vi "Image in Header or Footer.vi"(0 "report in":refnum<class "NI_HTML.lvclass">, 5 "select header or footer":u16(ring) items=["Left Header", "Left Footer", "Center Header", "Center Footer", "Right Herader", "Right Footer"], 9 "image path":string, 11 "error in (no error)":errorcluster, 12 "text above image":string) -> (4 "report out":refnum<class "NI_HTML.lvclass">, 15 "error out":errorcluster)   [LabVIEW 2017, in "NI_HTML.lvclass"]
doc: "This VI sets an image for the report header or footer.\n\nRemember, with the HTML report type the left, center, and right header texts are placed on separate lines."
uses:
  <vilib>/Utility/NIReport.llb/HTML/NI_HTML.lvclass
  <vilib>/Utility/NIReport.llb/HTML/NI_HTML.lvclass/NI_HTML.ctl
  <vilib>/Utility/NIReport.llb/NI_ReportGenerationCore.lvlib
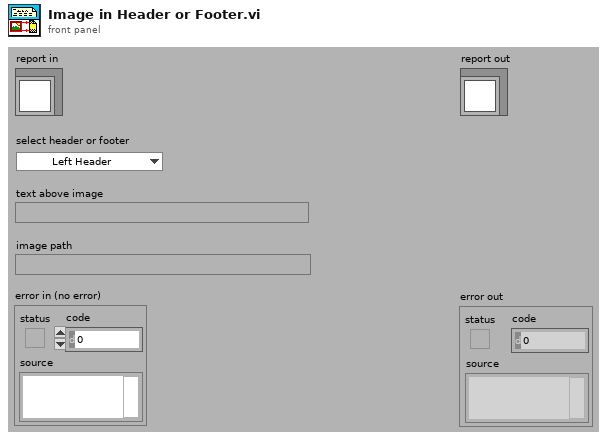
[diagram p1: front panel]
types:
  T1 = typedef "NI_ReportGenerationCore.lvlib/HTML Report Data.ctl" = cluster{"Body Text":string, "Font Tag":string, "Title Text":string, "Header Text":string, "Footer Text":string, "Image List":path[]}
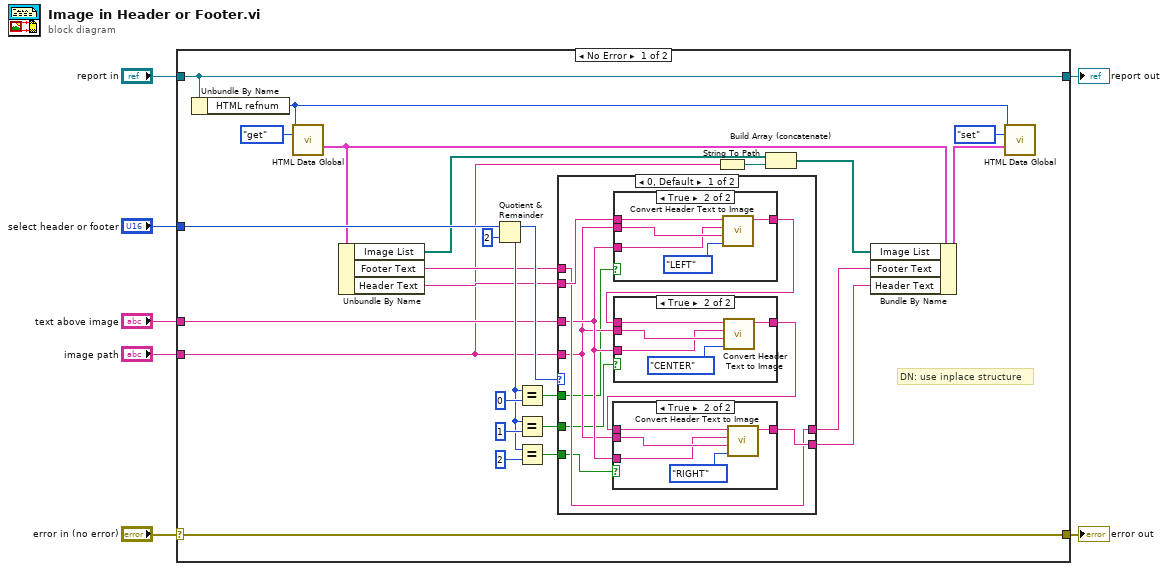
[diagram p0: block diagram]
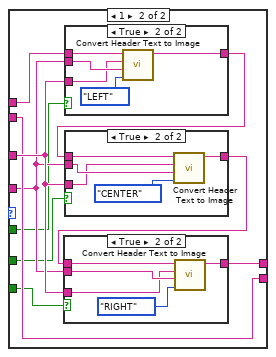
[diagram p5: hidden frame]
diagram:
  n1 = case shown="No Error" "error in (no error)" {
    selector: "error in (no error)" -> [w33 w91]
    tunnel: [w33 w91] -> w6
    tunnel: [w11 w90] -> w4
    tunnel: "report in" -> [w11 w90]
    tunnel: "select header or footer" -> [w18 _]
    tunnel: "text above image" -> [w17 _]
    tunnel: "image path" -> [w16 _]
    frame No Error {
      # "DN: use inplace structure"
      n2 = Unbundle By Name(w11) -> ("HTML refnum"=w8:u32)
      n3 = call <vilib>:"HTML Data Global.vi"("HTML refnum"=w8, "menu"=enum16{"init", "get", "set", "delete"}."get") -> ("HTML report data out"=w13:T1)  [unwired: 1 in, 12 out]
      n4 = Unbundle By Name(w13) -> ("Image List"=w14:path[], "Footer Text"=w19:string, "Header Text"=w21:string)
      n5 = Quotient & Remainder(x=w18, y=u8 2) -> (x-y*floor(x/y)=w24:u16, floor(x/y)=w25:u16)
      n6 = Equal?(x=w25, y=u16 0) -> (x = y?=w29:bool)
      n7 = Equal?(x=w25, y=u16 1) -> (x = y?=w30:bool)
      n8 = Equal?(x=w25, y=u16 2) -> (x = y?=w31:bool)
      n9 = case shown="0, Default" w24 {
        tunnel: [w39 w67] -> w20
        tunnel: w19 -> [w39 w66]
        tunnel: w21 -> [w41 w68]
        tunnel: [w40 w68] -> w22
        tunnel: w17 -> [w38 w69]
        tunnel: w16 -> [w37 w65]
        tunnel: w29 -> [w36 w64]
        tunnel: w30 -> [w35 w63]
        tunnel: w31 -> [w34 w62]
        frame 0, Default {
          n10 = case shown="True" w36 {
            tunnel: [w56 w61] -> w43
            tunnel: w41 -> [w56 w60]
            tunnel: w38 -> [_ w58]
            tunnel: w37 -> [_ w59]
            frame False {
            }
            frame True {
              n11 = call <vilib>:"Convert Header Text to Image.vi"("Enum"=enum16{"LEFT", "CENTER", "RIGHT"}."LEFT", "image path"=w59, "text above image"=w58, "HTML In"=w60) -> ("HTML Out"=w61:string)  [unwired: 7 out]
            }
          }
          n12 = case shown="True" w35 {
            tunnel: [w50 w55] -> w42
            tunnel: w43 -> [w50 w54]
            tunnel: w38 -> [_ w52]
            tunnel: w37 -> [_ w53]
            frame False {
            }
            frame True {
              n13 = call <vilib>:"Convert Header Text to Image.vi"("Enum"=enum16{"LEFT", "CENTER", "RIGHT"}."CENTER", "image path"=w53, "text above image"=w52, "HTML In"=w54) -> ("HTML Out"=w55:string)  [unwired: 7 out]
            }
          }
          n14 = case shown="True" w34 {
            tunnel: [w44 w49] -> w40
            tunnel: w42 -> [w44 w48]
            tunnel: w38 -> [_ w46]
            tunnel: w37 -> [_ w47]
            frame False {
            }
            frame True {
              n15 = call <vilib>:"Convert Header Text to Image.vi"("Enum"=enum16{"LEFT", "CENTER", "RIGHT"}."RIGHT", "image path"=w47, "text above image"=w46, "HTML In"=w48) -> ("HTML Out"=w49:string)  [unwired: 7 out]
            }
          }
        }
        frame 1 {
          n16 = case shown="True" w64 {
            tunnel: [w84 w85] -> w71
            tunnel: w66 -> [w84 w89]
            tunnel: w69 -> [_ w87]
            tunnel: w65 -> [_ w88]
            frame False {
            }
            frame True {
              n17 = call <vilib>:"Convert Header Text to Image.vi"("Enum"=enum16{"LEFT", "CENTER", "RIGHT"}."LEFT", "image path"=w88, "text above image"=w87, "HTML In"=w89) -> ("HTML Out"=w85:string)  [unwired: 7 out]
            }
          }
          n18 = case shown="True" w63 {
            tunnel: [w78 w83] -> w70
            tunnel: w71 -> [w78 w82]
            tunnel: w69 -> [_ w79]
            tunnel: w65 -> [_ w81]
            frame False {
            }
            frame True {
              n19 = call <vilib>:"Convert Header Text to Image.vi"("Enum"=enum16{"LEFT", "CENTER", "RIGHT"}."CENTER", "image path"=w81, "text above image"=w79, "HTML In"=w82) -> ("HTML Out"=w83:string)  [unwired: 7 out]
            }
          }
          n20 = case shown="True" w62 {
            tunnel: [w72 w77] -> w67
            tunnel: w70 -> [w72 w76]
            tunnel: w69 -> [_ w74]
            tunnel: w65 -> [_ w75]
            frame False {
            }
            frame True {
              n21 = call <vilib>:"Convert Header Text to Image.vi"("Enum"=enum16{"LEFT", "CENTER", "RIGHT"}."RIGHT", "image path"=w75, "text above image"=w74, "HTML In"=w76) -> ("HTML Out"=w77:string)  [unwired: 7 out]
            }
          }
        }
      }
      n22 = String To Path(string=w16) -> (path=w32:path)
      n23 = Build Array (concatenate)(w14, w32) -> (w12:path[])
      n24 = Bundle By Name(cluster=w13, "Image List"=w12, "Footer Text"=w20, "Header Text"=w22) -> (w9:T1)
      n25 = call <vilib>:"HTML Data Global.vi"("HTML refnum"=w8, "menu"=enum16{"init", "get", "set", "delete"}."set", "HTML report data in"=w9) -> ()  [unwired: 13 out]
    }
    frame Error {
    }
  }
  "error out" <- w6
  "report out" <- w4
